vi "VIItem.vi"(7 "Selection Type":refnum<class "MGI_SelectionType.lvclass"> caption="Selection Type (Click)", 10 "error in (no error)":errorcluster, 11 "Text":string) -> (2 "error out":errorcluster, 3 "VIItem Item":refnum<data-value>)   [LabVIEW 2016, in "MGI_VIItem.lvclass"]
doc: "VIItem Constructor. In addition to the standard MenuItem Fields/functionality, a VIItem has the following available through Propery Nodes:\nshort-cut\n\nIf a VIItem is used in a menu for a menu type other than VI, it is treated as a regular MenuItem\n\nAuthored by Derek E. Trepanier\nsupport@mooregoodideas.com\nwww.mooregoodideas.com\n\nCopyright (c) 2012, Moore Good Ideas, Inc.\n\nAll rights reserved.\n\nRedistribution and use in source and binary forms, with or without modification, are permitted provided that the following conditions are met:\n\n * Redistributions of source code must retain the above copyright notice, this list of conditions and the following disclaimer.\n * Redistributions in binary form must reproduce the above copyright notice, this list of conditions and the following disclaimer in the documentation and/or other materials provided with the distribution.\n * Neither the name of Moore Good Ideas, Inc. nor the names of its contributors may be used to endorse or promote products derived from this software without specific prior written permission.\n\nTHIS SOFTWARE IS PROVIDED BY THE COPYRIGHT HOLDERS AND CONTRIBUTORS \"AS IS\" AND ANY EXPRESS OR IMPLIED WARRANTIES, INCLUDING, BUT NOT LIMITED TO, THE IMPLIED WARRANTIES OF MERCHANTABILITY AND FITNESS FOR A PARTICULAR PURPOSE ARE DISCLAIMED. IN NO EVENT SHALL THE COPYRIGHT OWNER OR CONTRIBUTORS BE LIABLE FOR ANY DIRECT, INDIRECT, INCIDENTAL, SPECIAL, EXEMPLARY, OR CONSEQUENTIAL DAMAGES (INCLUDING, BUT NOT LIMITED TO, PROCUREMENT OF SUBSTITUTE GOODS OR SERVICES; LOSS OF USE, DATA, OR PROFITS; OR BUSINESS INTERRUPTION) HOWEVER CAUSED AND ON ANY THEORY OF LIABILITY, WHETHER IN CONTRACT, STRICT LIABILITY, OR TORT (INCLUDING NEGLIGENCE OR OTHERWISE) ARISING IN ANY WAY OUT OF THE USE OF THIS SOFTWARE, EVEN IF ADVISED OF THE POSSIBILITY OF SUCH DAMAGE."
uses:
  <userlib>/_MGI/Menu Building/MenuItem/VIItem/MGI_VIItem.lvclass
  C:/Program Files (x86)/National Instruments/LabVIEW 2016/user.lib/_MGI/Menu Building/MenuItem/MGI_MenuItem.lvclass
  <userlib>/_MGI/Menu Building/SelectionType/MGI_SelectionType.lvclass
  <userlib>/_MGI/Menu Building/MenuItem/MGI_MenuItem.lvclass
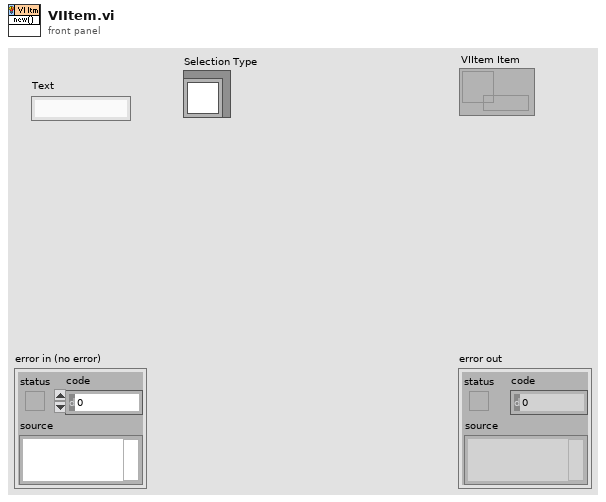
[diagram p1: front panel]
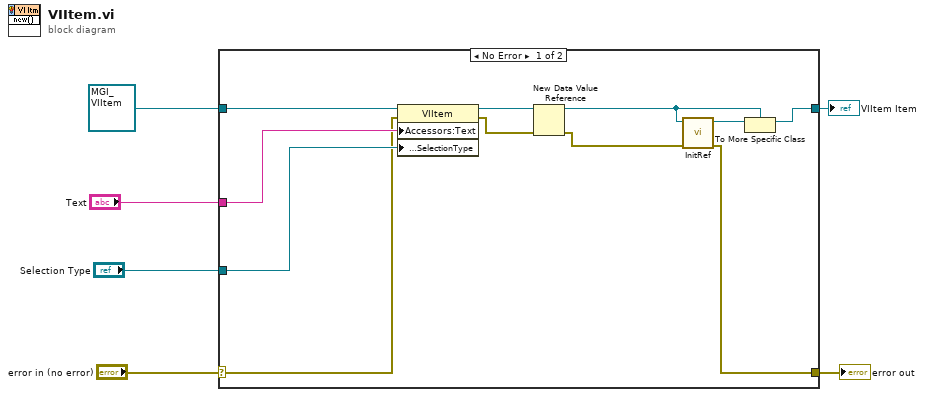
[diagram p0: block diagram]
diagram:
  n1 = case shown="No Error" "error in (no error)" {
    selector: "error in (no error)" -> [w13 w18]
    tunnel: [w7 w18] -> w5
    tunnel: refnum<class "MGI_VIItem.lvclass"> refnum ("MenubarItem in") -> [w17 _]
    tunnel: [w9 _] -> w3
    tunnel: "Text" -> [w15 _]
    tunnel: "Selection Type" -> [w14 _]
    frame No Error {
      n2 = property class="VIItem"(reference=w17, error in=w13, "Accessors:Text"=w15, "Accessors:SelectionType"=w14) -> (reference out=w16:refnum<class "MGI_VIItem.lvclass">, error out=w12:errorcluster)
      n3 = New Data Value Reference(data value=w16, error in=w12) -> (data value reference=w8:refnum<data-value>, error out=w10:errorcluster)
      n4 = call <userlib>:"InitRef.vi"("error in (no error)"=w10, "MenuItem in"=w8) -> ("error out"=w7:errorcluster, "MenuItem out"=w11:refnum<data-value>)  [unwired: 8 in]
      n5 = To More Specific Class(target class=w8, reference=w11) -> (specific class reference=w9:refnum<data-value>)  [unwired: 1 in, 1 out]
    }
    frame Error {
    }
  }
  "error out" <- w5
  "VIItem Item" <- w3
